vi "make_installer_exe.vi"(4 "config_value":T2, 6 "config_include":T1, 8 "error in (no error)":errorcluster, 10 "installer_directory":path, 11 "setup_filename in":path) -> (0 "error out":errorcluster, 3 "setup_filename out":path)   [LabVIEW 2015, in "lv-bin-7zip.lvlib"]
uses:
  lv-bin-7zip.lvlib
  public/api/v1/_controls/config_value.ctl
  public/api/v1/_controls/config_include.ctl
  <userlib>/antonio-alexander/lv-bin/public/api/v1/v1.lvlib
  public/api/v1/v1.lvlib
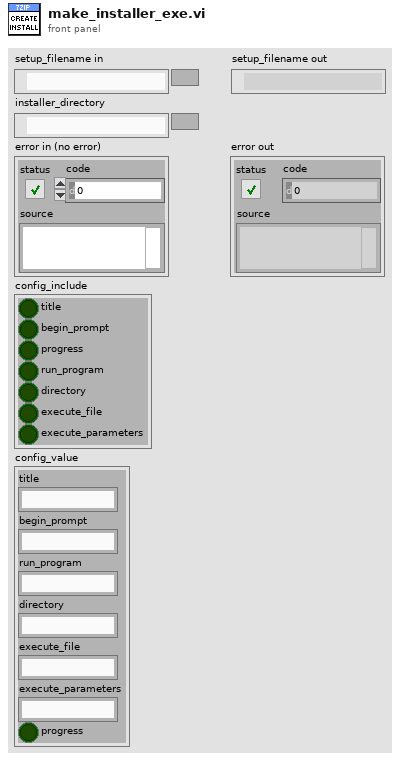
[diagram p1: front panel]
types:
  T1 = typedef "lv-bin-7zip.lvlib/v1.lvlib/config_include.ctl" = cluster{"title":bool, "begin_prompt":bool, "progress":bool, "run_program":bool, "directory":bool, "execute_file":bool, "execute_parameters":bool}
  T2 = typedef "lv-bin-7zip.lvlib/v1.lvlib/config_value.ctl" = cluster{"title":string, "begin_prompt":string, "run_program":string, "directory":string, "execute_file":string, "execute_parameters":string, "progress":bool}
  T3 = typedef "lv-bin.lvlib/v1.lvlib/temp_dir_config.ctl" = cluster{"root_folder":path, "prefix":string}
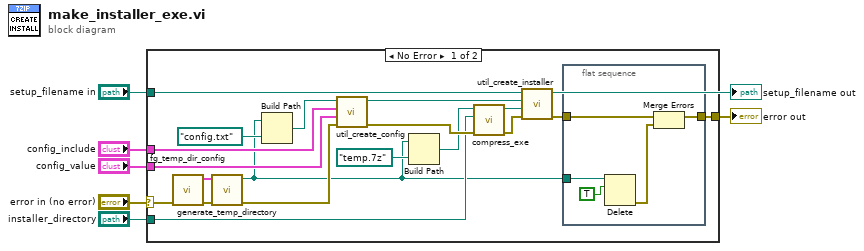
[diagram p0: block diagram]
diagram:
  n1 = case shown="No Error" "error in (no error)" {
    selector: "error in (no error)" -> [w9 w31]
    tunnel: "installer_directory" -> [w21 _]
    tunnel: "setup_filename in" -> [w14 _]
    tunnel: [w12 w31] -> w2
    tunnel: "config_include" -> [w16 _]
    tunnel: "config_value" -> [w15 _]
    frame No Error {
      n2 = call "fg_temp_dir_config.vi"("error in (no error)"=w9) -> ("error out"=w10:errorcluster, "temp_dir_config out"=w11:T3)  [unwired: 9 in]
      n3 = call <userlib>:"generate_temp_directory.vi"("error in (no error)"=w10, "configuration"=w11) -> ("error out"=w24:errorcluster, "temp_dir"=w7:path)  [unwired: 8 in]
      n4 = Build Path(base path=w7, name or relative path=path "config.txt" ("Path in (Relative)")) -> (appended path=w8:path)
      n5 = call "util_create_config.vi"("error in (no error)"=w24, "config_value"=w15, "config_include"=w16, "config_file in"=w8) -> ("error out"=w25:errorcluster, "config_file out"=w18:path)  [unwired: 6 in]
      n6 = Build Path(base path=w7, name or relative path=path "temp.7z" ("Path in (Relative)")) -> (appended path=w22:path)
      n7 = call "compress_exe.vi"("error in (no error)"=w25, "files_to_add"=w21, "archive_path in"=w22) -> ("error out"=w19:errorcluster, "archive_path out"=w17:path)  [unwired: 7 in]
      n8 = call "util_create_installer.vi"("error in (no error)"=w19, "archive"=w17, "config"=w18, "install_file in"=w14) -> ("error out"=w13:errorcluster)  [unwired: 6 in, 1 out]
      n9 = flat-sequence {
        tunnel: w7 -> [w30]
        tunnel: w13 -> [w28]
        tunnel: [w26] -> w12
        frame #0 {
          n10 = Delete(path (use dialog)=w30, entire hierarchy (F)=TRUE) -> (error out=w27:errorcluster)  [unwired: 3 in, 2 out]
          n11 = Merge Errors(w28, w27) -> (w26:errorcluster)
        }
      }
    }
    frame Error {
    }
  }
  "error out" <- w2
  "setup_filename out" <- "setup_filename in"
